vi "Get ProtoParser DLL Directory.vi"() -> (0 "Proto Parser Directory":path)   [LabVIEW 2024, in "gRPC Template Creation Utility.lvlib"]
uses:
  gRPC Template Creation Utility.lvlib
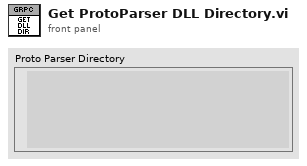
[diagram p1: front panel]
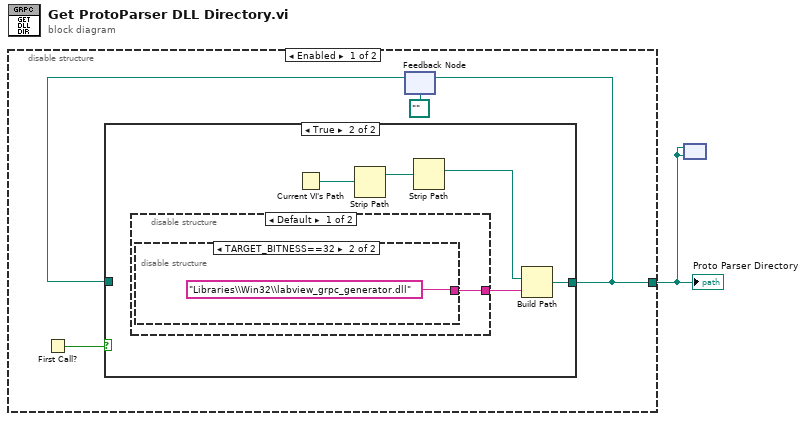
[diagram p0: block diagram]
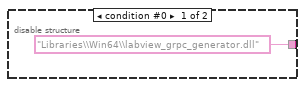
[diagram p3: hidden frame]
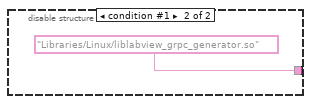
[diagram p4: hidden frame]
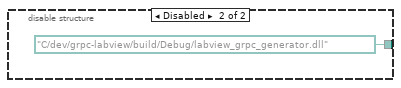
[diagram p5: hidden frame]
diagram:
  n1 = disable-structure shown="Enabled" {
    disable-tunnel: [w4 path "C:/dev/grpc-labview/build/Debug/labview_grpc_generator.dll" ("Proto Parser Directory")] -> w1
    frame Enabled {
      n2 = First Call?() -> (First Call?: T/F=w5:bool)
      n3 = feedback #1(path "" ("appended path")) -> (w3:path)
      n4 = case shown="True" w5 {
        tunnel: [w6 w7] -> w4
        tunnel: w3 -> [w6 _]
        frame False {
        }
        frame True {
          n5 = disable-structure shown="Default" {
            disable-tunnel: [w12 "Libraries/Linux/liblabview_grpc_generator.so" ("name or relative path")] -> w8
            frame condition #0 (active) {
              n6 = disable-structure shown="TARGET_BITNESS==32" {
                disable-tunnel: ["Libraries\\Win64\\labview_grpc_generator.dll" ("name or relative path") "Libraries\\Win32\\labview_grpc_generator.dll" ("name or relative path")] -> w12
                frame condition #0 {
                }
                frame condition #1 (active) {
                }
              }
            }
            frame condition #1 {
            }
          }
          n7 = Current VI's Path() -> (path=w9:path)
          n8 = Strip Path(path=w9) -> (stripped path=w10:path)  [unwired: 1 out]
          n9 = Strip Path(path=w10) -> (stripped path=w11:path)  [unwired: 1 out]
          n10 = Build Path(base path=w11, name or relative path=w8) -> (appended path=w7:path)
        }
      }
      n11 = feedback-in #1(w4) -> ()
    }
    frame Disabled {
    }
  }
  "Proto Parser Directory" <- w1
  n12 = node(w1, w1) -> ()  [unwired: 1 out]
